vi "Set Position.vi"(8 "error in (no error)":errorcluster, 10 "Position":dbl, 11 "Device Manager in":refnum<class "Device Manager.lvclass">) -> (0 "error out":errorcluster, 3 "Device Manager out":refnum<class "Device Manager.lvclass">)   [LabVIEW 2020, in "Device Manager.lvlib" / "Device Manager.lvclass"]
uses:
  Device Manager.lvclass
  Device Manager.lvclass/Device Manager.ctl
  Motor/Motor Messages/Set Position Msg/Set Position Msg.lvclass
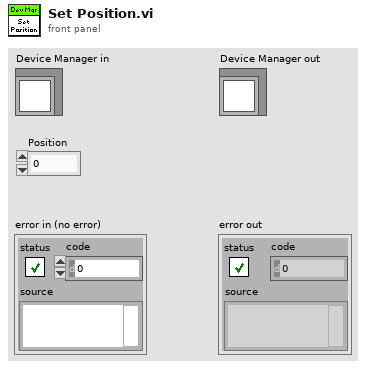
[diagram p1: front panel]
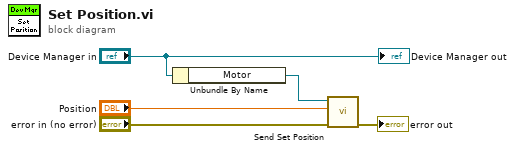
[diagram p0: block diagram]
diagram:
  n1 = Unbundle By Name("Device Manager in") -> ("Motor"=w4:refnum<class "Message Enqueuer.lvclass">)
  n2 = call "Send Set Position.vi"("error in (no error)"="error in (no error)", "Position"="Position", "Message Enqueuer"=w4) -> ("error out"=→"error out":errorcluster)  [unwired: 7 in, 1 out]
  "Device Manager out" <- "Device Manager in"
